vi "windowClose.vi"(8 "error in (no error)":errorcluster, 11 "BuildWorker in":refnum<class "BuildWorker.lvclass">) -> (0 "error out":errorcluster, 2 "Discard?":bool, 3 "Actor wUI out":refnum<class "Actor wUI.lvclass">)   [LabVIEW 2017, in "BuildWorker.lvlib" / "BuildWorker.lvclass"]
uses:
  BuildWorker.lvclass
  C:/Users/Public/Documents/wc/BuildFarm/src/LabVIEW/vi.lib/BenjaminR/Build Farm/Actors/Framework/Actor wUI/Actor wUI.lvclass
  C:/Program Files (x86)/National Instruments/LabVIEW 2017/vi.lib/ActorFramework/Actor/Actor.lvclass
  Framework/Actor wUI/Actor wUI.lvclass
  <vilib>/ActorFramework/Actor/Actor.lvclass/Actor.ctl
  <vilib>/ActorFramework/Message Enqueuer/Message Enqueuer.lvclass/Message Enqueuer.ctl
  <vilib>/ActorFramework/Message Enqueuer/Init from Existing Queue.vi
  <vilib>/ActorFramework/Message Enqueuer/Enqueue.vi
  Framework/Actor wUI Messages/Hide UI Msg/Hide UI Msg.lvclass
  C:/Program Files (x86)/National Instruments/LabVIEW 2017/vi.lib/ActorFramework/Message/Message.lvclass
  <vilib>/ActorFramework/Message Priority Queue/Priority Enqueue.vi
  <vilib>/ActorFramework/Message Enqueuer/Message Enqueuer.lvclass
  <vilib>/ActorFramework/Actor/Actor.lvclass
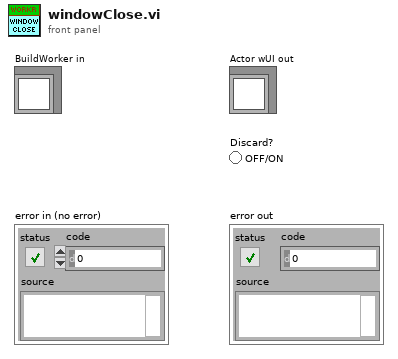
[diagram p1: front panel]
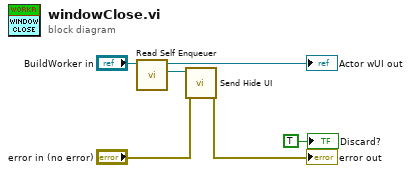
[diagram p0: block diagram]
diagram:
  n1 = call <vilib>:"Read Self Enqueuer.vi"("Actor"="BuildWorker in") -> ("Self Enqueuer"=w3:refnum<class "Message Enqueuer.lvclass">)  [unwired: 10 in]
  n2 = call "Send Hide UI.vi"("error in (no error)"="error in (no error)", "Message Enqueuer in"=w3) -> ("error out"=→"error out":errorcluster)  [unwired: 8 in, 1 out]
  "Actor wUI out" <- "BuildWorker in"
  "Discard?" <- TRUE ("Discard?")
